vi "Untitled 1.vi"() -> ()   [LabVIEW 2015]
uses:
  <vilib>/Analysis/1siggen.llb/Ramp Pattern by Delta.vi
  <vilib>/Analysis/NI_AALBase.lvlib
panel:
  out "Ramp Pattern":dbl[](array[numeric])
  in  "Cluster":T1
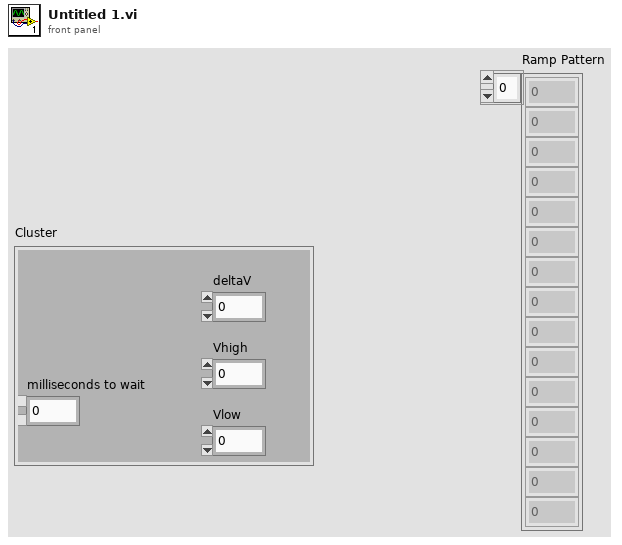
[diagram p1: front panel]
types:
  T1 = cluster{"milliseconds to wait":u32, "deltaV":dbl, "Vhigh":dbl, "Vlow":dbl}
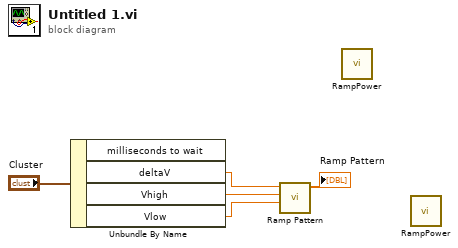
[diagram p0: block diagram]
diagram:
  n1 = Unbundle By Name("Cluster") -> ("deltaV"=w4:dbl, "Vhigh"=w3:dbl, "Vlow"=w2:dbl)  [unwired: 1 out]
  n2 = call-poly <vilib>:"Ramp Pattern.vi"("start"=w2, "end"=w3, "delta"=w4) -> ("Ramp Pattern"=→"Ramp Pattern":dbl[])  [unwired: 6 in, 2 out]
  n3 = call "RampPower.vi"() -> ()  [unwired: 9 in, 3 out]
  n4 = call "RampPower.vi"() -> ()  [unwired: 9 in, 3 out]
